vi "Experiment 13.vi"() -> ()   [LabVIEW 2026]
doc: "Experiment 13\nThis experiment is like Experiment 12 but contains only 4 parallel loops (instead of 10 as in Exp 12)."
uses:
  <vilib>/AdvancedString/1D String Array to Delimited String (string).vi
  <vilib>/Analysis/baseanly.llb/Mean (DBL).vi
  <vilib>/Analysis/NI_AALBase.lvlib
panel:
  out "No. Of Iterations As Block Of Text (easy to copy into Excel)":string
  out "No. Of Iterations Executed - Loop 4":i32
  out "Output - Loop 4":dbl[](array[numeric]) format="%.3f"
  out "No. Of Iterations Executed - Loop 3":i32
  out "Output - Loop 3":dbl[](array[numeric]) format="%.3f"
  out "Avg. No. Of Iterations Executed - All Loops":dbl format="%.1f"
  out "No. Of Iterations Executed - Loop 2":i32
  out "Output - Loop 2":dbl[](array[numeric]) format="%.3f"
  out "No. Of Iterations Executed - Loop 1":i32
  out "Output - Loop 1":dbl[](array[numeric]) format="%.3f"
  out "Stop VI?":bool
  # "Experiment 13"
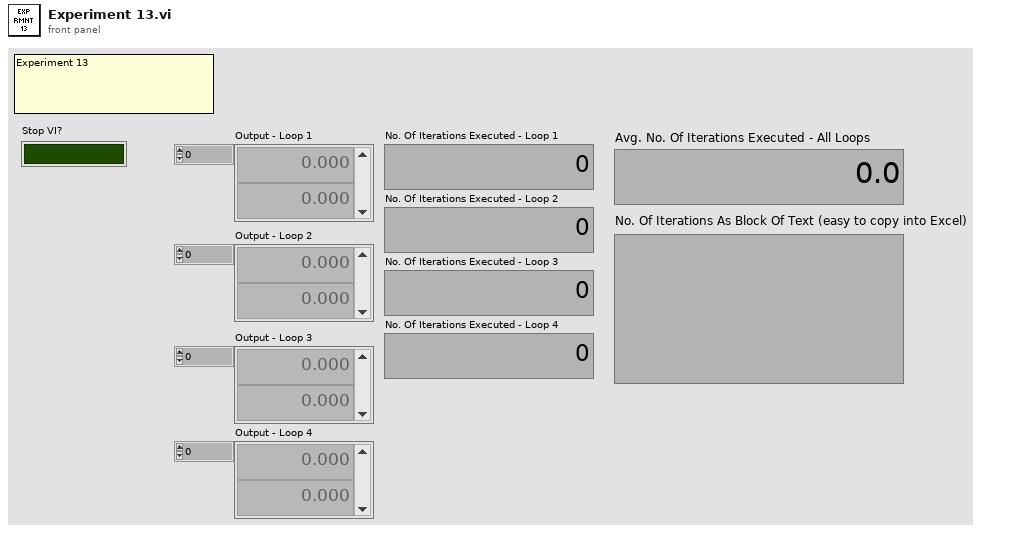
[diagram p1: front panel]
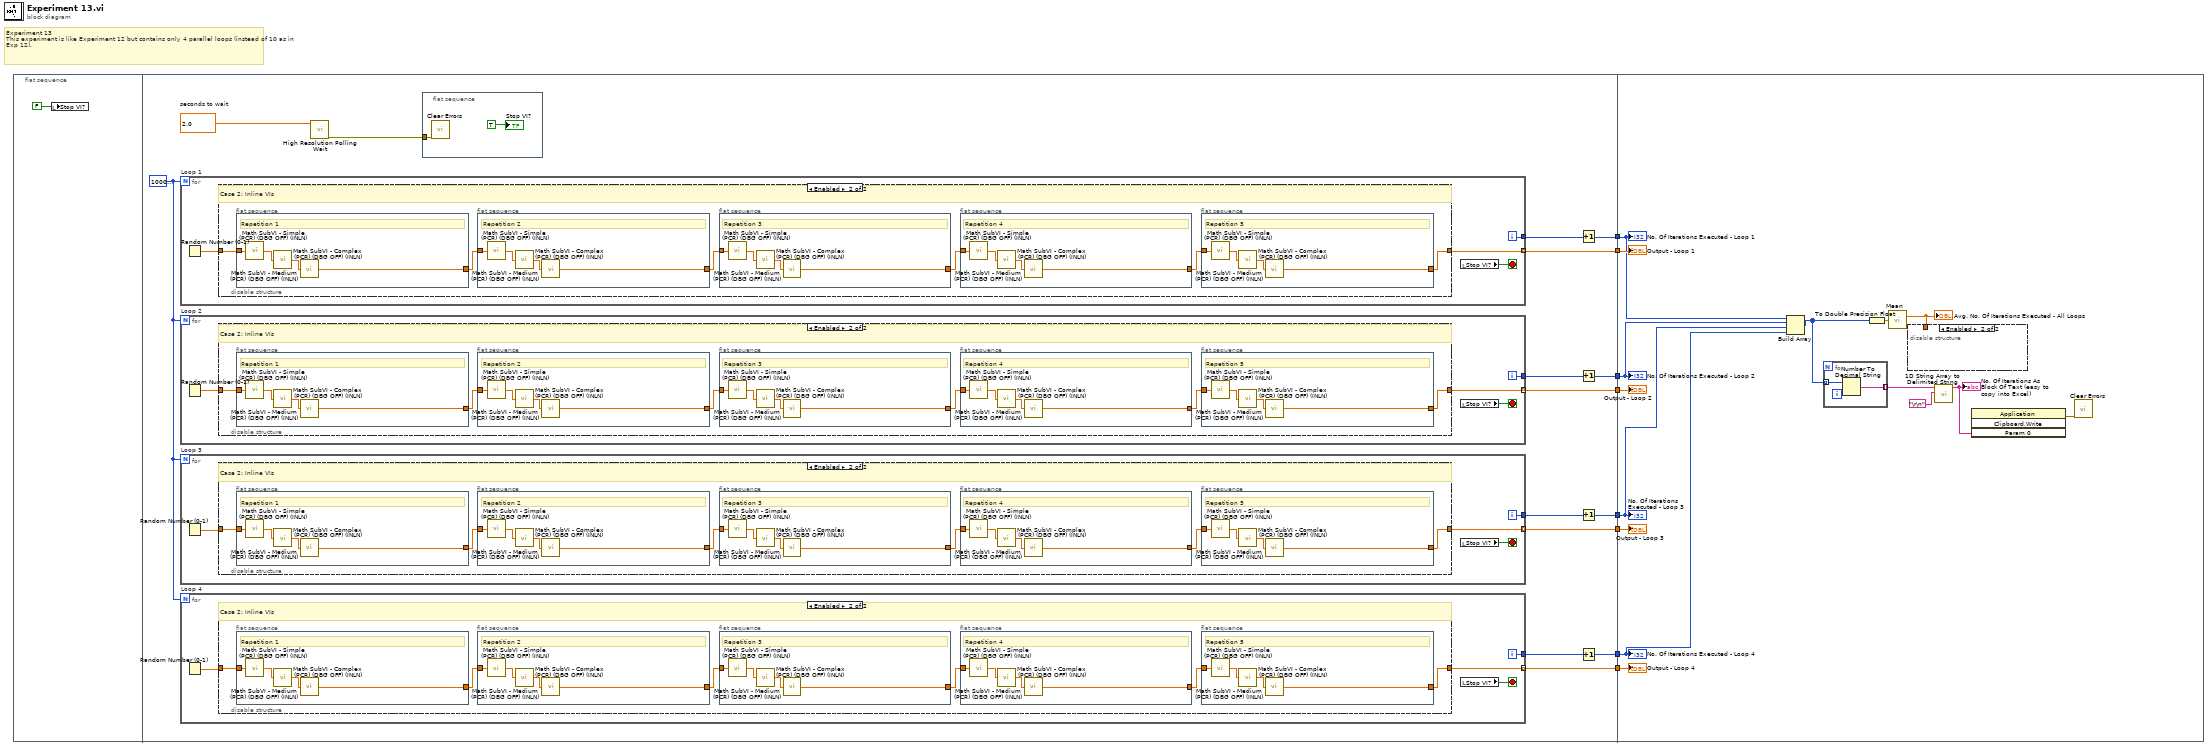
[diagram p0: block diagram]
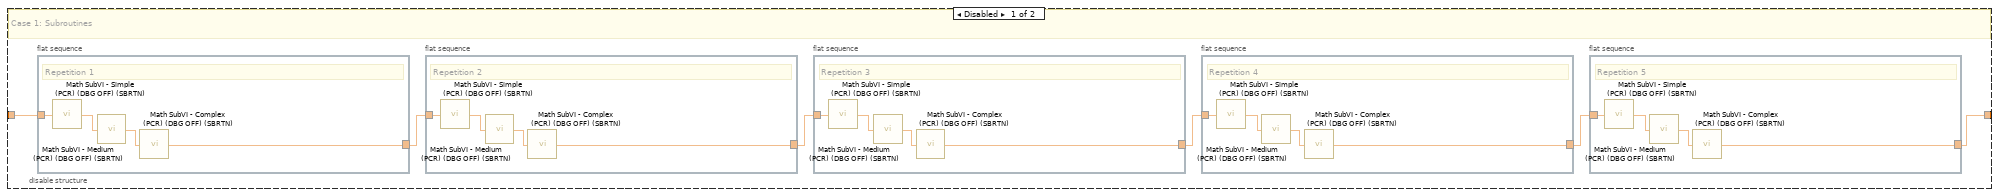
[diagram p2: hidden frame]
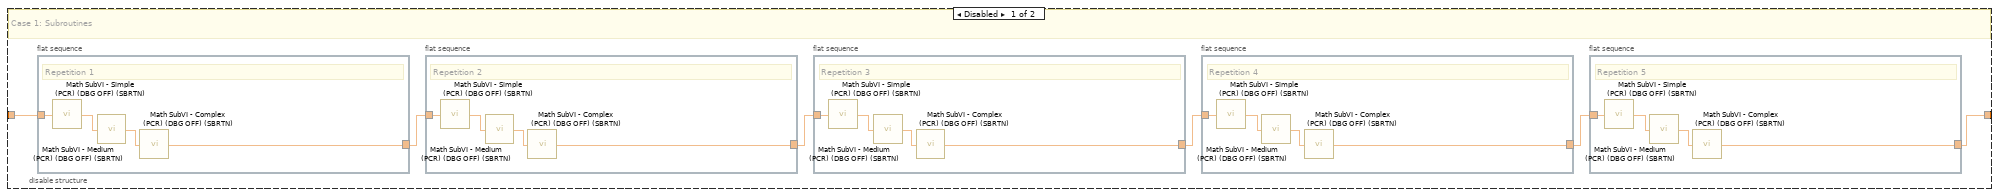
[diagram p3: hidden frame]
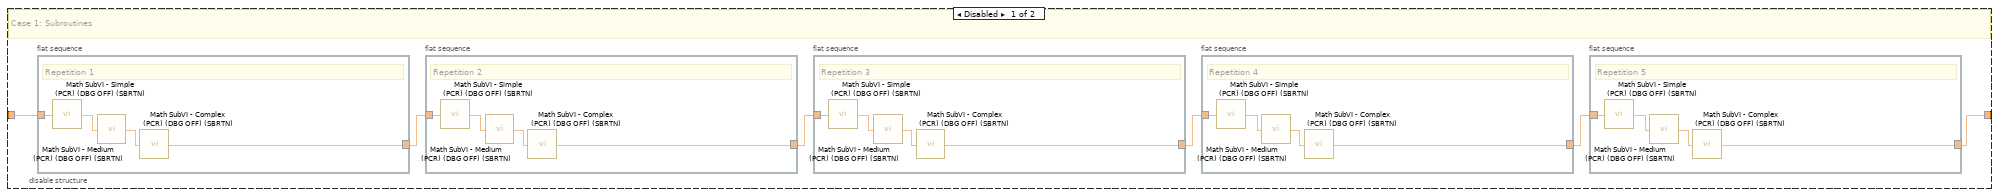
[diagram p4: hidden frame]
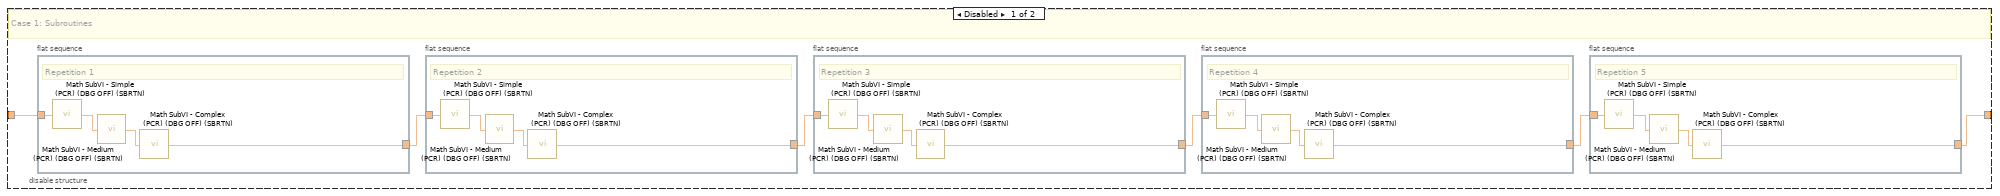
[diagram p5: hidden frame]
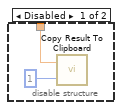
[diagram p6: hidden frame]
diagram:
  # "Experiment 13\nThis experiment is like Experiment 12 but contains only 4 parallel loops (instead of 10 as in Exp 12)."
  n1 = flat-sequence {
    tunnel: [w22] -> w8
    tunnel: [w20] -> w7
    tunnel: [w19] -> w6
    tunnel: [w16] -> w5
    tunnel: [w18] -> w4
    tunnel: [w14] -> w3
    tunnel: [w12] -> w2
    tunnel: [w17] -> w1
    tunnel: w8 -> [w265]
    tunnel: w7 -> [w263]
    tunnel: w6 -> [w262]
    tunnel: w5 -> [w264]
    tunnel: w4 -> [w258]
    tunnel: w3 -> [w260]
    tunnel: w2 -> [w259]
    tunnel: w1 -> [w257]
    frame #0 {
      n2 = local write "Stop VI?"(FALSE) -> ()
    }
    frame #1 {
      w10 = 10000000
      w24 = 2.0  # seconds to wait
      n3 = for "Loop 1" {
        N: w10 -> [_]
        tunnel: [w196] -> w22 mode=indexing
        tunnel: [w197] -> w21
        i -> [w197]
        stop <- w198 stop-if-true
        n4 = Random Number (0-1)() -> (number: 0 to 1=w195:dbl)
        n5 = disable-structure shown="Enabled" {
          disable-tunnel: w195 -> [w204 w230]
          disable-tunnel: [w203 w225] -> w196
          frame Disabled {
            # "Case 1: Subroutines"
            n6 = flat-sequence {
              tunnel: w204 -> [w224]
              tunnel: [w221] -> w199
              frame #0 {
                # "Repetition 1"
                n7 = call "Math SubVI - Simple (PCR) (DBG OFF) (SBRTN).vi"("Input"=w224) -> ("Output"=w222:dbl)
                n8 = call "Math SubVI - Medium (PCR) (DBG OFF) (SBRTN).vi"("Input"=w222) -> ("Output"=w223:dbl)
                n9 = call "Math SubVI - Complex (PCR) (DBG OFF) (SBRTN).vi"("Input"=w223) -> ("Output"=w221:dbl)
              }
            }
            n10 = flat-sequence {
              tunnel: w199 -> [w220]
              tunnel: [w217] -> w202
              frame #0 {
                # "Repetition 2"
                n11 = call "Math SubVI - Simple (PCR) (DBG OFF) (SBRTN).vi"("Input"=w220) -> ("Output"=w218:dbl)
                n12 = call "Math SubVI - Medium (PCR) (DBG OFF) (SBRTN).vi"("Input"=w218) -> ("Output"=w219:dbl)
                n13 = call "Math SubVI - Complex (PCR) (DBG OFF) (SBRTN).vi"("Input"=w219) -> ("Output"=w217:dbl)
              }
            }
            n14 = flat-sequence {
              tunnel: w202 -> [w216]
              tunnel: [w213] -> w201
              frame #0 {
                # "Repetition 3"
                n15 = call "Math SubVI - Simple (PCR) (DBG OFF) (SBRTN).vi"("Input"=w216) -> ("Output"=w214:dbl)
                n16 = call "Math SubVI - Medium (PCR) (DBG OFF) (SBRTN).vi"("Input"=w214) -> ("Output"=w215:dbl)
                n17 = call "Math SubVI - Complex (PCR) (DBG OFF) (SBRTN).vi"("Input"=w215) -> ("Output"=w213:dbl)
              }
            }
            n18 = flat-sequence {
              tunnel: w201 -> [w212]
              tunnel: [w209] -> w200
              frame #0 {
                # "Repetition 4"
                n19 = call "Math SubVI - Simple (PCR) (DBG OFF) (SBRTN).vi"("Input"=w212) -> ("Output"=w210:dbl)
                n20 = call "Math SubVI - Medium (PCR) (DBG OFF) (SBRTN).vi"("Input"=w210) -> ("Output"=w211:dbl)
                n21 = call "Math SubVI - Complex (PCR) (DBG OFF) (SBRTN).vi"("Input"=w211) -> ("Output"=w209:dbl)
              }
            }
            n22 = flat-sequence {
              tunnel: w200 -> [w208]
              tunnel: [w205] -> w203
              frame #0 {
                # "Repetition 5"
                n23 = call "Math SubVI - Simple (PCR) (DBG OFF) (SBRTN).vi"("Input"=w208) -> ("Output"=w206:dbl)
                n24 = call "Math SubVI - Medium (PCR) (DBG OFF) (SBRTN).vi"("Input"=w206) -> ("Output"=w207:dbl)
                n25 = call "Math SubVI - Complex (PCR) (DBG OFF) (SBRTN).vi"("Input"=w207) -> ("Output"=w205:dbl)
              }
            }
          }
          frame Enabled {
            # "Case 2: Inline VIs"
            n26 = flat-sequence {
              tunnel: w230 -> [w250]
              tunnel: [w247] -> w229
              frame #0 {
                # "Repetition 1"
                n27 = call "Math SubVI - Simple (PCR) (DBG OFF) (INLN).vi"("Input"=w250) -> ("Output"=w248:dbl)
                n28 = call "Math SubVI - Medium (PCR) (DBG OFF) (INLN).vi"("Input"=w248) -> ("Output"=w249:dbl)
                n29 = call "Math SubVI - Complex (PCR) (DBG OFF) (INLN).vi"("Input"=w249) -> ("Output"=w247:dbl)
              }
            }
            n30 = flat-sequence {
              tunnel: w229 -> [w246]
              tunnel: [w243] -> w228
              frame #0 {
                # "Repetition 2"
                n31 = call "Math SubVI - Simple (PCR) (DBG OFF) (INLN).vi"("Input"=w246) -> ("Output"=w244:dbl)
                n32 = call "Math SubVI - Medium (PCR) (DBG OFF) (INLN).vi"("Input"=w244) -> ("Output"=w245:dbl)
                n33 = call "Math SubVI - Complex (PCR) (DBG OFF) (INLN).vi"("Input"=w245) -> ("Output"=w243:dbl)
              }
            }
            n34 = flat-sequence {
              tunnel: w228 -> [w242]
              tunnel: [w239] -> w227
              frame #0 {
                # "Repetition 3"
                n35 = call "Math SubVI - Simple (PCR) (DBG OFF) (INLN).vi"("Input"=w242) -> ("Output"=w240:dbl)
                n36 = call "Math SubVI - Medium (PCR) (DBG OFF) (INLN).vi"("Input"=w240) -> ("Output"=w241:dbl)
                n37 = call "Math SubVI - Complex (PCR) (DBG OFF) (INLN).vi"("Input"=w241) -> ("Output"=w239:dbl)
              }
            }
            n38 = flat-sequence {
              tunnel: w227 -> [w238]
              tunnel: [w235] -> w226
              frame #0 {
                # "Repetition 4"
                n39 = call "Math SubVI - Simple (PCR) (DBG OFF) (INLN).vi"("Input"=w238) -> ("Output"=w236:dbl)
                n40 = call "Math SubVI - Medium (PCR) (DBG OFF) (INLN).vi"("Input"=w236) -> ("Output"=w237:dbl)
                n41 = call "Math SubVI - Complex (PCR) (DBG OFF) (INLN).vi"("Input"=w237) -> ("Output"=w235:dbl)
              }
            }
            n42 = flat-sequence {
              tunnel: w226 -> [w234]
              tunnel: [w231] -> w225
              frame #0 {
                # "Repetition 5"
                n43 = call "Math SubVI - Simple (PCR) (DBG OFF) (INLN).vi"("Input"=w234) -> ("Output"=w232:dbl)
                n44 = call "Math SubVI - Medium (PCR) (DBG OFF) (INLN).vi"("Input"=w232) -> ("Output"=w233:dbl)
                n45 = call "Math SubVI - Complex (PCR) (DBG OFF) (INLN).vi"("Input"=w233) -> ("Output"=w231:dbl)
              }
            }
          }
        }
        n46 = local read "Stop VI?"() -> (w198:bool)
      }
      n47 = for "Loop 2" {
        N: w10 -> [_]
        tunnel: [w140] -> w16 mode=indexing
        tunnel: [w141] -> w15
        i -> [w141]
        stop <- w142 stop-if-true
        n48 = Random Number (0-1)() -> (number: 0 to 1=w139:dbl)
        n49 = disable-structure shown="Enabled" {
          disable-tunnel: w139 -> [w148 w174]
          disable-tunnel: [w147 w169] -> w140
          frame Disabled {
            # "Case 1: Subroutines"
            n50 = flat-sequence {
              tunnel: w148 -> [w168]
              tunnel: [w165] -> w143
              frame #0 {
                # "Repetition 1"
                n51 = call "Math SubVI - Simple (PCR) (DBG OFF) (SBRTN).vi"("Input"=w168) -> ("Output"=w166:dbl)
                n52 = call "Math SubVI - Medium (PCR) (DBG OFF) (SBRTN).vi"("Input"=w166) -> ("Output"=w167:dbl)
                n53 = call "Math SubVI - Complex (PCR) (DBG OFF) (SBRTN).vi"("Input"=w167) -> ("Output"=w165:dbl)
              }
            }
            n54 = flat-sequence {
              tunnel: w143 -> [w164]
              tunnel: [w161] -> w146
              frame #0 {
                # "Repetition 2"
                n55 = call "Math SubVI - Simple (PCR) (DBG OFF) (SBRTN).vi"("Input"=w164) -> ("Output"=w162:dbl)
                n56 = call "Math SubVI - Medium (PCR) (DBG OFF) (SBRTN).vi"("Input"=w162) -> ("Output"=w163:dbl)
                n57 = call "Math SubVI - Complex (PCR) (DBG OFF) (SBRTN).vi"("Input"=w163) -> ("Output"=w161:dbl)
              }
            }
            n58 = flat-sequence {
              tunnel: w146 -> [w160]
              tunnel: [w157] -> w145
              frame #0 {
                # "Repetition 3"
                n59 = call "Math SubVI - Simple (PCR) (DBG OFF) (SBRTN).vi"("Input"=w160) -> ("Output"=w158:dbl)
                n60 = call "Math SubVI - Medium (PCR) (DBG OFF) (SBRTN).vi"("Input"=w158) -> ("Output"=w159:dbl)
                n61 = call "Math SubVI - Complex (PCR) (DBG OFF) (SBRTN).vi"("Input"=w159) -> ("Output"=w157:dbl)
              }
            }
            n62 = flat-sequence {
              tunnel: w145 -> [w156]
              tunnel: [w153] -> w144
              frame #0 {
                # "Repetition 4"
                n63 = call "Math SubVI - Simple (PCR) (DBG OFF) (SBRTN).vi"("Input"=w156) -> ("Output"=w154:dbl)
                n64 = call "Math SubVI - Medium (PCR) (DBG OFF) (SBRTN).vi"("Input"=w154) -> ("Output"=w155:dbl)
                n65 = call "Math SubVI - Complex (PCR) (DBG OFF) (SBRTN).vi"("Input"=w155) -> ("Output"=w153:dbl)
              }
            }
            n66 = flat-sequence {
              tunnel: w144 -> [w152]
              tunnel: [w149] -> w147
              frame #0 {
                # "Repetition 5"
                n67 = call "Math SubVI - Simple (PCR) (DBG OFF) (SBRTN).vi"("Input"=w152) -> ("Output"=w150:dbl)
                n68 = call "Math SubVI - Medium (PCR) (DBG OFF) (SBRTN).vi"("Input"=w150) -> ("Output"=w151:dbl)
                n69 = call "Math SubVI - Complex (PCR) (DBG OFF) (SBRTN).vi"("Input"=w151) -> ("Output"=w149:dbl)
              }
            }
          }
          frame Enabled {
            # "Case 2: Inline VIs"
            n70 = flat-sequence {
              tunnel: w174 -> [w194]
              tunnel: [w191] -> w173
              frame #0 {
                # "Repetition 1"
                n71 = call "Math SubVI - Simple (PCR) (DBG OFF) (INLN).vi"("Input"=w194) -> ("Output"=w192:dbl)
                n72 = call "Math SubVI - Medium (PCR) (DBG OFF) (INLN).vi"("Input"=w192) -> ("Output"=w193:dbl)
                n73 = call "Math SubVI - Complex (PCR) (DBG OFF) (INLN).vi"("Input"=w193) -> ("Output"=w191:dbl)
              }
            }
            n74 = flat-sequence {
              tunnel: w173 -> [w190]
              tunnel: [w187] -> w172
              frame #0 {
                # "Repetition 2"
                n75 = call "Math SubVI - Simple (PCR) (DBG OFF) (INLN).vi"("Input"=w190) -> ("Output"=w188:dbl)
                n76 = call "Math SubVI - Medium (PCR) (DBG OFF) (INLN).vi"("Input"=w188) -> ("Output"=w189:dbl)
                n77 = call "Math SubVI - Complex (PCR) (DBG OFF) (INLN).vi"("Input"=w189) -> ("Output"=w187:dbl)
              }
            }
            n78 = flat-sequence {
              tunnel: w172 -> [w186]
              tunnel: [w183] -> w171
              frame #0 {
                # "Repetition 3"
                n79 = call "Math SubVI - Simple (PCR) (DBG OFF) (INLN).vi"("Input"=w186) -> ("Output"=w184:dbl)
                n80 = call "Math SubVI - Medium (PCR) (DBG OFF) (INLN).vi"("Input"=w184) -> ("Output"=w185:dbl)
                n81 = call "Math SubVI - Complex (PCR) (DBG OFF) (INLN).vi"("Input"=w185) -> ("Output"=w183:dbl)
              }
            }
            n82 = flat-sequence {
              tunnel: w171 -> [w182]
              tunnel: [w179] -> w170
              frame #0 {
                # "Repetition 4"
                n83 = call "Math SubVI - Simple (PCR) (DBG OFF) (INLN).vi"("Input"=w182) -> ("Output"=w180:dbl)
                n84 = call "Math SubVI - Medium (PCR) (DBG OFF) (INLN).vi"("Input"=w180) -> ("Output"=w181:dbl)
                n85 = call "Math SubVI - Complex (PCR) (DBG OFF) (INLN).vi"("Input"=w181) -> ("Output"=w179:dbl)
              }
            }
            n86 = flat-sequence {
              tunnel: w170 -> [w178]
              tunnel: [w175] -> w169
              frame #0 {
                # "Repetition 5"
                n87 = call "Math SubVI - Simple (PCR) (DBG OFF) (INLN).vi"("Input"=w178) -> ("Output"=w176:dbl)
                n88 = call "Math SubVI - Medium (PCR) (DBG OFF) (INLN).vi"("Input"=w176) -> ("Output"=w177:dbl)
                n89 = call "Math SubVI - Complex (PCR) (DBG OFF) (INLN).vi"("Input"=w177) -> ("Output"=w175:dbl)
              }
            }
          }
        }
        n90 = local read "Stop VI?"() -> (w142:bool)
      }
      n91 = for "Loop 3" {
        N: w10 -> [_]
        tunnel: [w84] -> w14 mode=indexing
        tunnel: [w85] -> w13
        i -> [w85]
        stop <- w86 stop-if-true
        n92 = Random Number (0-1)() -> (number: 0 to 1=w83:dbl)
        n93 = disable-structure shown="Enabled" {
          disable-tunnel: w83 -> [w92 w118]
          disable-tunnel: [w91 w113] -> w84
          frame Disabled {
            # "Case 1: Subroutines"
            n94 = flat-sequence {
              tunnel: w92 -> [w112]
              tunnel: [w109] -> w87
              frame #0 {
                # "Repetition 1"
                n95 = call "Math SubVI - Simple (PCR) (DBG OFF) (SBRTN).vi"("Input"=w112) -> ("Output"=w110:dbl)
                n96 = call "Math SubVI - Medium (PCR) (DBG OFF) (SBRTN).vi"("Input"=w110) -> ("Output"=w111:dbl)
                n97 = call "Math SubVI - Complex (PCR) (DBG OFF) (SBRTN).vi"("Input"=w111) -> ("Output"=w109:dbl)
              }
            }
            n98 = flat-sequence {
              tunnel: w87 -> [w108]
              tunnel: [w105] -> w90
              frame #0 {
                # "Repetition 2"
                n99 = call "Math SubVI - Simple (PCR) (DBG OFF) (SBRTN).vi"("Input"=w108) -> ("Output"=w106:dbl)
                n100 = call "Math SubVI - Medium (PCR) (DBG OFF) (SBRTN).vi"("Input"=w106) -> ("Output"=w107:dbl)
                n101 = call "Math SubVI - Complex (PCR) (DBG OFF) (SBRTN).vi"("Input"=w107) -> ("Output"=w105:dbl)
              }
            }
            n102 = flat-sequence {
              tunnel: w90 -> [w104]
              tunnel: [w101] -> w89
              frame #0 {
                # "Repetition 3"
                n103 = call "Math SubVI - Simple (PCR) (DBG OFF) (SBRTN).vi"("Input"=w104) -> ("Output"=w102:dbl)
                n104 = call "Math SubVI - Medium (PCR) (DBG OFF) (SBRTN).vi"("Input"=w102) -> ("Output"=w103:dbl)
                n105 = call "Math SubVI - Complex (PCR) (DBG OFF) (SBRTN).vi"("Input"=w103) -> ("Output"=w101:dbl)
              }
            }
            n106 = flat-sequence {
              tunnel: w89 -> [w100]
              tunnel: [w97] -> w88
              frame #0 {
                # "Repetition 4"
                n107 = call "Math SubVI - Simple (PCR) (DBG OFF) (SBRTN).vi"("Input"=w100) -> ("Output"=w98:dbl)
                n108 = call "Math SubVI - Medium (PCR) (DBG OFF) (SBRTN).vi"("Input"=w98) -> ("Output"=w99:dbl)
                n109 = call "Math SubVI - Complex (PCR) (DBG OFF) (SBRTN).vi"("Input"=w99) -> ("Output"=w97:dbl)
              }
            }
            n110 = flat-sequence {
              tunnel: w88 -> [w96]
              tunnel: [w93] -> w91
              frame #0 {
                # "Repetition 5"
                n111 = call "Math SubVI - Simple (PCR) (DBG OFF) (SBRTN).vi"("Input"=w96) -> ("Output"=w94:dbl)
                n112 = call "Math SubVI - Medium (PCR) (DBG OFF) (SBRTN).vi"("Input"=w94) -> ("Output"=w95:dbl)
                n113 = call "Math SubVI - Complex (PCR) (DBG OFF) (SBRTN).vi"("Input"=w95) -> ("Output"=w93:dbl)
              }
            }
          }
          frame Enabled {
            # "Case 2: Inline VIs"
            n114 = flat-sequence {
              tunnel: w118 -> [w138]
              tunnel: [w135] -> w117
              frame #0 {
                # "Repetition 1"
                n115 = call "Math SubVI - Simple (PCR) (DBG OFF) (INLN).vi"("Input"=w138) -> ("Output"=w136:dbl)
                n116 = call "Math SubVI - Medium (PCR) (DBG OFF) (INLN).vi"("Input"=w136) -> ("Output"=w137:dbl)
                n117 = call "Math SubVI - Complex (PCR) (DBG OFF) (INLN).vi"("Input"=w137) -> ("Output"=w135:dbl)
              }
            }
            n118 = flat-sequence {
              tunnel: w117 -> [w134]
              tunnel: [w131] -> w116
              frame #0 {
                # "Repetition 2"
                n119 = call "Math SubVI - Simple (PCR) (DBG OFF) (INLN).vi"("Input"=w134) -> ("Output"=w132:dbl)
                n120 = call "Math SubVI - Medium (PCR) (DBG OFF) (INLN).vi"("Input"=w132) -> ("Output"=w133:dbl)
                n121 = call "Math SubVI - Complex (PCR) (DBG OFF) (INLN).vi"("Input"=w133) -> ("Output"=w131:dbl)
              }
            }
            n122 = flat-sequence {
              tunnel: w116 -> [w130]
              tunnel: [w127] -> w115
              frame #0 {
                # "Repetition 3"
                n123 = call "Math SubVI - Simple (PCR) (DBG OFF) (INLN).vi"("Input"=w130) -> ("Output"=w128:dbl)
                n124 = call "Math SubVI - Medium (PCR) (DBG OFF) (INLN).vi"("Input"=w128) -> ("Output"=w129:dbl)
                n125 = call "Math SubVI - Complex (PCR) (DBG OFF) (INLN).vi"("Input"=w129) -> ("Output"=w127:dbl)
              }
            }
            n126 = flat-sequence {
              tunnel: w115 -> [w126]
              tunnel: [w123] -> w114
              frame #0 {
                # "Repetition 4"
                n127 = call "Math SubVI - Simple (PCR) (DBG OFF) (INLN).vi"("Input"=w126) -> ("Output"=w124:dbl)
                n128 = call "Math SubVI - Medium (PCR) (DBG OFF) (INLN).vi"("Input"=w124) -> ("Output"=w125:dbl)
                n129 = call "Math SubVI - Complex (PCR) (DBG OFF) (INLN).vi"("Input"=w125) -> ("Output"=w123:dbl)
              }
            }
            n130 = flat-sequence {
              tunnel: w114 -> [w122]
              tunnel: [w119] -> w113
              frame #0 {
                # "Repetition 5"
                n131 = call "Math SubVI - Simple (PCR) (DBG OFF) (INLN).vi"("Input"=w122) -> ("Output"=w120:dbl)
                n132 = call "Math SubVI - Medium (PCR) (DBG OFF) (INLN).vi"("Input"=w120) -> ("Output"=w121:dbl)
                n133 = call "Math SubVI - Complex (PCR) (DBG OFF) (INLN).vi"("Input"=w121) -> ("Output"=w119:dbl)
              }
            }
          }
        }
        n134 = local read "Stop VI?"() -> (w86:bool)
      }
      n135 = for "Loop 4" {
        N: w10 -> [_]
        tunnel: [w28] -> w12 mode=indexing
        tunnel: [w29] -> w11
        i -> [w29]
        stop <- w30 stop-if-true
        n136 = Random Number (0-1)() -> (number: 0 to 1=w27:dbl)
        n137 = disable-structure shown="Enabled" {
          disable-tunnel: w27 -> [w36 w62]
          disable-tunnel: [w35 w57] -> w28
          frame Disabled {
            # "Case 1: Subroutines"
            n138 = flat-sequence {
              tunnel: w36 -> [w56]
              tunnel: [w53] -> w31
              frame #0 {
                # "Repetition 1"
                n139 = call "Math SubVI - Simple (PCR) (DBG OFF) (SBRTN).vi"("Input"=w56) -> ("Output"=w54:dbl)
                n140 = call "Math SubVI - Medium (PCR) (DBG OFF) (SBRTN).vi"("Input"=w54) -> ("Output"=w55:dbl)
                n141 = call "Math SubVI - Complex (PCR) (DBG OFF) (SBRTN).vi"("Input"=w55) -> ("Output"=w53:dbl)
              }
            }
            n142 = flat-sequence {
              tunnel: w31 -> [w52]
              tunnel: [w49] -> w34
              frame #0 {
                # "Repetition 2"
                n143 = call "Math SubVI - Simple (PCR) (DBG OFF) (SBRTN).vi"("Input"=w52) -> ("Output"=w50:dbl)
                n144 = call "Math SubVI - Medium (PCR) (DBG OFF) (SBRTN).vi"("Input"=w50) -> ("Output"=w51:dbl)
                n145 = call "Math SubVI - Complex (PCR) (DBG OFF) (SBRTN).vi"("Input"=w51) -> ("Output"=w49:dbl)
              }
            }
            n146 = flat-sequence {
              tunnel: w34 -> [w48]
              tunnel: [w45] -> w33
              frame #0 {
                # "Repetition 3"
                n147 = call "Math SubVI - Simple (PCR) (DBG OFF) (SBRTN).vi"("Input"=w48) -> ("Output"=w46:dbl)
                n148 = call "Math SubVI - Medium (PCR) (DBG OFF) (SBRTN).vi"("Input"=w46) -> ("Output"=w47:dbl)
                n149 = call "Math SubVI - Complex (PCR) (DBG OFF) (SBRTN).vi"("Input"=w47) -> ("Output"=w45:dbl)
              }
            }
            n150 = flat-sequence {
              tunnel: w33 -> [w44]
              tunnel: [w41] -> w32
              frame #0 {
                # "Repetition 4"
                n151 = call "Math SubVI - Simple (PCR) (DBG OFF) (SBRTN).vi"("Input"=w44) -> ("Output"=w42:dbl)
                n152 = call "Math SubVI - Medium (PCR) (DBG OFF) (SBRTN).vi"("Input"=w42) -> ("Output"=w43:dbl)
                n153 = call "Math SubVI - Complex (PCR) (DBG OFF) (SBRTN).vi"("Input"=w43) -> ("Output"=w41:dbl)
              }
            }
            n154 = flat-sequence {
              tunnel: w32 -> [w40]
              tunnel: [w37] -> w35
              frame #0 {
                # "Repetition 5"
                n155 = call "Math SubVI - Simple (PCR) (DBG OFF) (SBRTN).vi"("Input"=w40) -> ("Output"=w38:dbl)
                n156 = call "Math SubVI - Medium (PCR) (DBG OFF) (SBRTN).vi"("Input"=w38) -> ("Output"=w39:dbl)
                n157 = call "Math SubVI - Complex (PCR) (DBG OFF) (SBRTN).vi"("Input"=w39) -> ("Output"=w37:dbl)
              }
            }
          }
          frame Enabled {
            # "Case 2: Inline VIs"
            n158 = flat-sequence {
              tunnel: w62 -> [w82]
              tunnel: [w79] -> w61
              frame #0 {
                # "Repetition 1"
                n159 = call "Math SubVI - Simple (PCR) (DBG OFF) (INLN).vi"("Input"=w82) -> ("Output"=w80:dbl)
                n160 = call "Math SubVI - Medium (PCR) (DBG OFF) (INLN).vi"("Input"=w80) -> ("Output"=w81:dbl)
                n161 = call "Math SubVI - Complex (PCR) (DBG OFF) (INLN).vi"("Input"=w81) -> ("Output"=w79:dbl)
              }
            }
            n162 = flat-sequence {
              tunnel: w61 -> [w78]
              tunnel: [w75] -> w60
              frame #0 {
                # "Repetition 2"
                n163 = call "Math SubVI - Simple (PCR) (DBG OFF) (INLN).vi"("Input"=w78) -> ("Output"=w76:dbl)
                n164 = call "Math SubVI - Medium (PCR) (DBG OFF) (INLN).vi"("Input"=w76) -> ("Output"=w77:dbl)
                n165 = call "Math SubVI - Complex (PCR) (DBG OFF) (INLN).vi"("Input"=w77) -> ("Output"=w75:dbl)
              }
            }
            n166 = flat-sequence {
              tunnel: w60 -> [w74]
              tunnel: [w71] -> w59
              frame #0 {
                # "Repetition 3"
                n167 = call "Math SubVI - Simple (PCR) (DBG OFF) (INLN).vi"("Input"=w74) -> ("Output"=w72:dbl)
                n168 = call "Math SubVI - Medium (PCR) (DBG OFF) (INLN).vi"("Input"=w72) -> ("Output"=w73:dbl)
                n169 = call "Math SubVI - Complex (PCR) (DBG OFF) (INLN).vi"("Input"=w73) -> ("Output"=w71:dbl)
              }
            }
            n170 = flat-sequence {
              tunnel: w59 -> [w70]
              tunnel: [w67] -> w58
              frame #0 {
                # "Repetition 4"
                n171 = call "Math SubVI - Simple (PCR) (DBG OFF) (INLN).vi"("Input"=w70) -> ("Output"=w68:dbl)
                n172 = call "Math SubVI - Medium (PCR) (DBG OFF) (INLN).vi"("Input"=w68) -> ("Output"=w69:dbl)
                n173 = call "Math SubVI - Complex (PCR) (DBG OFF) (INLN).vi"("Input"=w69) -> ("Output"=w67:dbl)
              }
            }
            n174 = flat-sequence {
              tunnel: w58 -> [w66]
              tunnel: [w63] -> w57
              frame #0 {
                # "Repetition 5"
                n175 = call "Math SubVI - Simple (PCR) (DBG OFF) (INLN).vi"("Input"=w66) -> ("Output"=w64:dbl)
                n176 = call "Math SubVI - Medium (PCR) (DBG OFF) (INLN).vi"("Input"=w64) -> ("Output"=w65:dbl)
                n177 = call "Math SubVI - Complex (PCR) (DBG OFF) (INLN).vi"("Input"=w65) -> ("Output"=w63:dbl)
              }
            }
          }
        }
        n178 = local read "Stop VI?"() -> (w30:bool)
      }
      n179 = call <vilib>:"High Resolution Polling Wait.vi"("seconds to wait"=w24) -> ("error out"=w23:errorcluster)  [unwired: 10 in]
      n180 = flat-sequence {
        tunnel: w23 -> [w25]
        frame #0 {
          n181 = call <vilib>:"Clear Errors.vi"("error in (no error)"=w25) -> ()  [unwired: 5 in, 2 out]
          "Stop VI?" <- TRUE
        }
      }
      n182 = Increment(x=w21) -> (x+1=w20:i32)
      n183 = Increment(x=w15) -> (x+1=w19:i32)
      n184 = Increment(x=w13) -> (x+1=w18:i32)
      n185 = Increment(x=w11) -> (x+1=w17:i32)
    }
    frame #2 {
      n186 = Build Array(w263, w262, w258, w257) -> (w255:i32[])
      n187 = for {
        tunnel: w255 -> [w269] mode=indexing
        tunnel: [w268] -> w254 mode=indexing
        n188 = Number To Decimal String(number=w269) -> (decimal integer string=w268:string)  [unwired: 1 in]
      }
      n189 = To Double Precision Float(number=w255) -> (double precision float=w256:dbl[])
      n190 = call-poly <vilib>:"Mean.vi"("X"=w256) -> ("mean"=w261:dbl)  [unwired: 1 out]
      "Avg. No. Of Iterations Executed - All Loops" <- w261
      n191 = disable-structure shown="Enabled" {
        disable-tunnel: w261 -> [w267 _]
        frame Disabled {
          n192 = call "Copy Result To Clipboard.vi"("No. Of Decimal Places (6)"=u32 1, "Input"=w267) -> ()
        }
        frame Enabled {
        }
      }
      n193 = call-poly <vilib>:"1D String Array to Delimited String.vi"("delimiter"="\r\n", "string array"=w254) -> ("delimited string"=w251:string)  [unwired: 9 in]
      "No. Of Iterations As Block Of Text (easy to copy into Excel)" <- w251
      n194 = invoke class="Application" method="Clipboard.Write"("Param 0"=w251) -> (error out=w252:errorcluster)  [unwired: 3 in, 3 out]
      n195 = call <vilib>:"Clear Errors.vi"("error in (no error)"=w252) -> ()  [unwired: 5 in, 2 out]
      "No. Of Iterations Executed - Loop 1" <- w263
      "Output - Loop 1" <- w265
      "No. Of Iterations Executed - Loop 2" <- w262
      "Output - Loop 2" <- w264
      "No. Of Iterations Executed - Loop 3" <- w258
      "Output - Loop 3" <- w260
      "No. Of Iterations Executed - Loop 4" <- w257
      "Output - Loop 4" <- w259
    }
  }
